vi "L10n.vi"(2 "Localize? (True)":bool=TRUE, 3 "String In":string) -> (1 "String Out":string)   [LabVIEW 2020, in "Set DDT Attributes.lvlib" / "Set DDT Properties.xnode"]
uses:
  <vilib>/express/express signal manip/GetorSetDDTAttributes/Set DDT Attributes/Set DDT Properties.xnode
panel:
  in  "Localized Strings":string[](array[string])
  in  "DNL_Strings":string[](array[string])
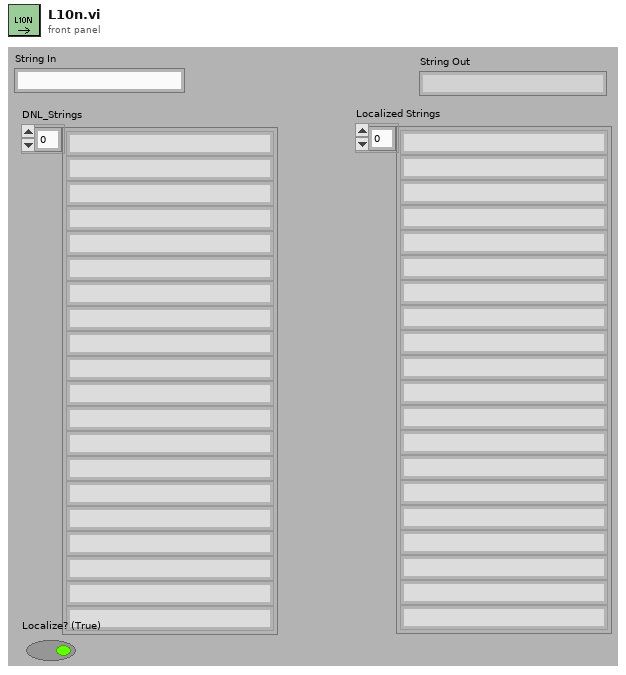
[diagram p1: front panel]
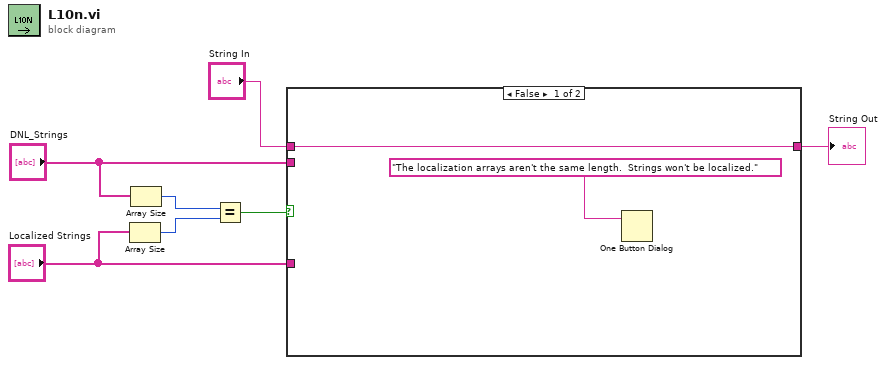
[diagram p0: block diagram]
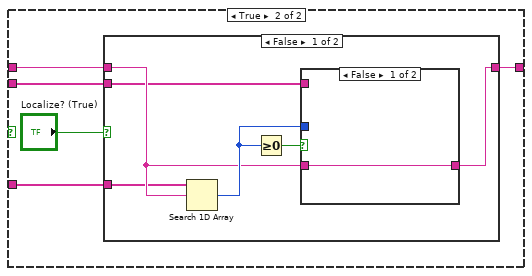
[diagram p2: hidden frame]
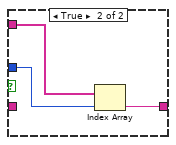
[diagram p3: hidden frame]
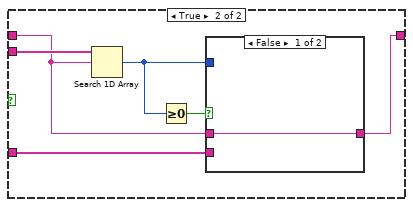
[diagram p4: hidden frame]
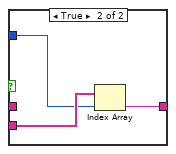
[diagram p5: hidden frame]
diagram:
  n1 = Array Size(array="Localized Strings") -> (size(s)=w6:i32)
  n2 = Array Size(array="DNL_Strings") -> (size(s)=w7:i32)
  n3 = Equal?(x=w7, y=w6) -> (x = y?=w5:bool)
  n4 = case shown="False" w5 {
    tunnel: "DNL_Strings" -> [_ w14]
    tunnel: "Localized Strings" -> [_ w13]
    tunnel: "String In" -> [w8 w11]
    tunnel: [w8 w12] -> w1
    frame False {
      n5 = One Button Dialog(message="The localization arrays aren't the same length.  Strings won't be localized.") -> ()  [unwired: 2 out]
    }
    frame True {
      n6 = case shown="False" "Localize? (True)" {
        tunnel: w14 -> [w15 w30]
        tunnel: w13 -> [w16 w27]
        tunnel: [w18 w26] -> w12
        tunnel: w11 -> [w17 w25]
        frame False {
          n7 = Search 1D Array(1D array=w16, element=w17) -> (index of element=w20:i32)  [unwired: 1 out]
          n8 = Greater Or Equal To 0?(x=w20) -> (x >= 0?=w19:bool)
          n9 = case shown="False" w19 {
            tunnel: w20 -> [_ w24]
            tunnel: [w21 w23] -> w18
            tunnel: w17 -> [w21 _]
            tunnel: w15 -> [_ w22]
            frame False {
            }
            frame True {
              n10 = Index Array(array=w22, index=w24) -> (element=w23:string)
            }
          }
        }
        frame True {
          n11 = Search 1D Array(1D array=w30, element=w25) -> (index of element=w29:i32)  [unwired: 1 out]
          n12 = Greater Or Equal To 0?(x=w29) -> (x >= 0?=w28:bool)
          n13 = case shown="False" w28 {
            tunnel: w29 -> [_ w33]
            tunnel: w27 -> [_ w34]
            tunnel: [w31 w32] -> w26
            tunnel: w25 -> [w31 _]
            frame False {
            }
            frame True {
              n14 = Index Array(array=w34, index=w33) -> (element=w32:string)
            }
          }
        }
      }
    }
  }
  "String Out" <- w1
